vi "Get Multiplier From Throttle.vi"(10 "Value from 1":dbl, 11 "Axis 3":dbl) -> (3 "Numeric":dbl)   [LabVIEW 2012]
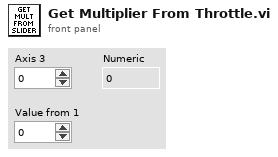
[diagram p1: front panel]
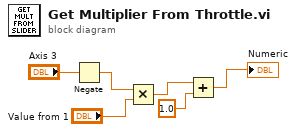
[diagram p0: block diagram]
diagram:
  n1 = Negate(x="Axis 3") -> (-x=w4:dbl)
  n2 = Multiply(x=w4, y="Value from 1") -> (x*y=w3:dbl)
  n3 = Add(x=w3, y=1.0) -> (x+y=→"Numeric":dbl)
